vi "New Button Gallery.vi"(8 "Error In":errorcluster) -> (0 "Error Out":errorcluster, 3 "New Button Gallery":refnum<class "QWidget.lvclass">)   [LabVIEW 2014]
doc: "Dynamically assembles a widget that contains a variety of push buttons, checkboxes, and radio buttons. These buttons/checkboxes are grouped within group boxes.\n\nThe caller must manually make the returned widget visible.\n\n\nCopyright (c) 2019 Sze Howe Koh.\nThis code is licensed under the MIT license."
uses:
  <vilib>/addons/LQ/Qt Widgets/QWidget/QWidget.lvclass
  <vilib>/addons/LQ/Qt Widgets/QBoxLayout/Direction.ctl
  <vilib>/addons/LQ/Qt Widgets/QGroupBox/setCheckable.vi
  <vilib>/addons/LQ/Qt Widgets/QGroupBox/QGroupBox.lvclass
  <vilib>/addons/LQ/Qt Widgets/QPushButton/QPushButton.lvclass
  <vilib>/addons/LQ/Qt Widgets/QBoxLayout/QBoxLayout.lvclass
  <vilib>/addons/LQ/Qt Widgets/QCheckBox/QCheckBox.lvclass
  <vilib>/addons/LQ/Qt Widgets/QRadioButton/QRadioButton.lvclass
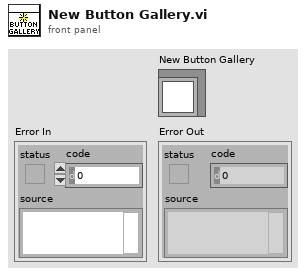
[diagram p1: front panel]
types:
  T1 = typedef "QBoxLayout.lvclass/Direction.ctl" = i32
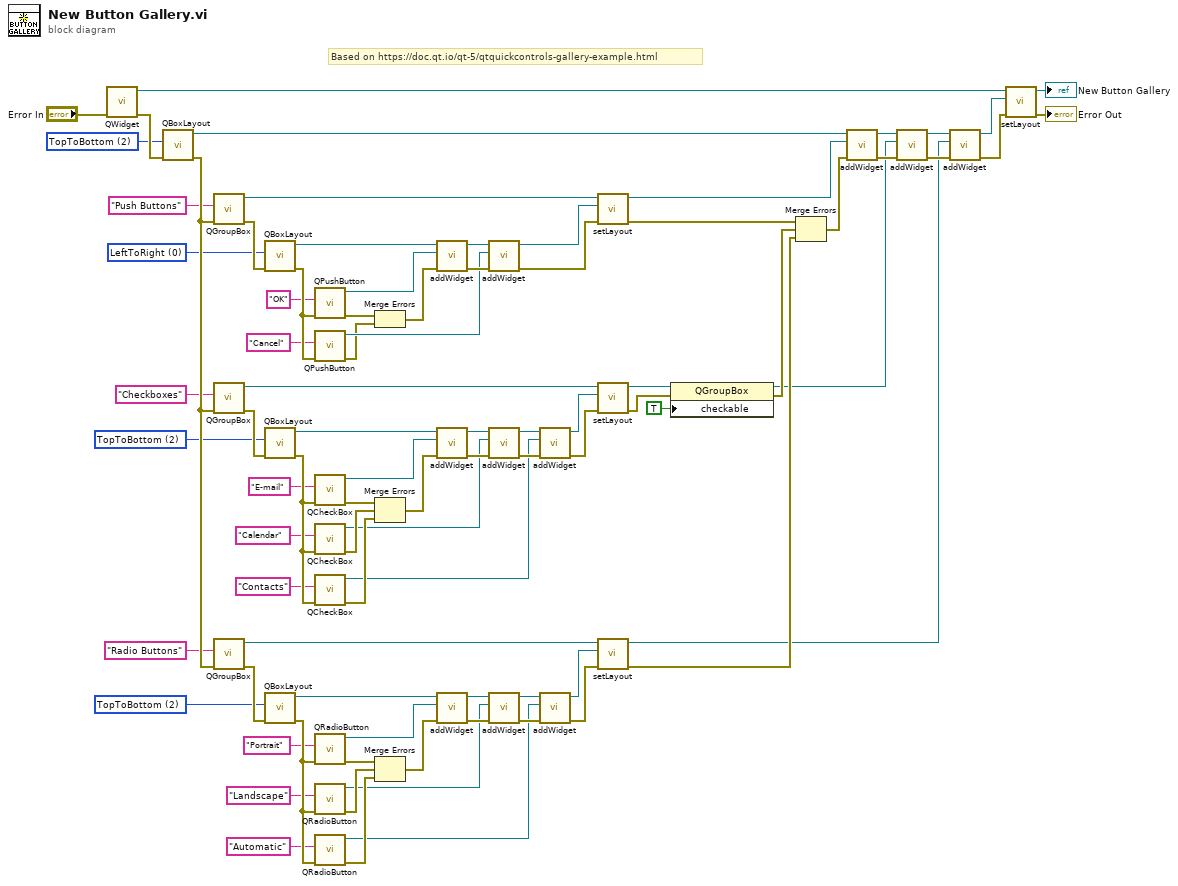
[diagram p0: block diagram]
diagram:
  w30 = T1 2 items=["LeftToRight", "RightToLeft", "TopToBottom", "BottomToTop"] ("direction")
  w44 = T1 2 items=["LeftToRight", "RightToLeft", "TopToBottom", "BottomToTop"] ("direction")
  w45 = T1 2 items=["LeftToRight", "RightToLeft", "TopToBottom", "BottomToTop"] ("direction")
  w46 = T1 0 items=["LeftToRight", "RightToLeft", "TopToBottom", "BottomToTop"] ("direction")
  # "Based on https://doc.qt.io/qt-5/qtquickcontrols-gallery-example.html"
  n1 = call <vilib>:"QWidget.vi"("Error In"="Error In") -> ("Error Out"=w83:errorcluster, "New QWidget"=w47:refnum<class "QWidget.lvclass">)  [unwired: 9 in]
  n2 = call <vilib>:"QBoxLayout.vi"("Error In"=w83, "direction"=w45) -> ("Error Out"=w75:errorcluster, "New QBoxLayout"=w49:refnum<class "QBoxLayout.lvclass">)  [unwired: 8 in]
  n3 = call <vilib>:"QGroupBox.vi"("Error In"=w75, "title"="Push Buttons") -> ("Error Out"=w84:errorcluster, "New QGroupBox"=w69:refnum<class "QGroupBox.lvclass">)  [unwired: 8 in]
  n4 = call <vilib>:"QGroupBox.vi"("Error In"=w75, "title"="Checkboxes") -> ("Error Out"=w77:errorcluster, "New QGroupBox"=w51:refnum<class "QGroupBox.lvclass">)  [unwired: 8 in]
  n5 = call <vilib>:"QGroupBox.vi"("Error In"=w75, "title"="Radio Buttons") -> ("Error Out"=w74:errorcluster, "New QGroupBox"=w14:refnum<class "QGroupBox.lvclass">)  [unwired: 8 in]
  n6 = call <vilib>:"QBoxLayout.vi"("Error In"=w84, "direction"=w46) -> ("Error Out"=w85:errorcluster, "New QBoxLayout"=w68:refnum<class "QBoxLayout.lvclass">)  [unwired: 8 in]
  n7 = call <vilib>:"QBoxLayout.vi"("Error In"=w77, "direction"=w44) -> ("Error Out"=w76:errorcluster, "New QBoxLayout"=w57:refnum<class "QBoxLayout.lvclass">)  [unwired: 8 in]
  n8 = call <vilib>:"QBoxLayout.vi"("Error In"=w74, "direction"=w30) -> ("Error Out"=w73:errorcluster, "New QBoxLayout"=w24:refnum<class "QBoxLayout.lvclass">)  [unwired: 8 in]
  n9 = call <vilib>:"QPushButton.vi"("Error In"=w85, "text"="OK") -> ("Error Out"=w42:errorcluster, "New QPushButton"=w66:refnum<class "QPushButton.lvclass">)  [unwired: 8 in]
  n10 = call <vilib>:"QPushButton.vi"("Error In"=w85, "text"="Cancel") -> ("Error Out"=w41:errorcluster, "New QPushButton"=w61:refnum<class "QPushButton.lvclass">)  [unwired: 8 in]
  n11 = call <vilib>:"QCheckBox.vi"("Error In"=w76, "text"="E-mail") -> ("Error Out"=w38:errorcluster, "New QCheckBox"=w54:refnum<class "QCheckBox.lvclass">)  [unwired: 8 in]
  n12 = call <vilib>:"QCheckBox.vi"("Error In"=w76, "text"="Calendar") -> ("Error Out"=w78:errorcluster, "New QCheckBox"=w53:refnum<class "QCheckBox.lvclass">)  [unwired: 8 in]
  n13 = call <vilib>:"QCheckBox.vi"("Error In"=w76, "text"="Contacts") -> ("Error Out"=w79:errorcluster, "New QCheckBox"=w52:refnum<class "QCheckBox.lvclass">)  [unwired: 8 in]
  n14 = call <vilib>:"QRadioButton.vi"("Error In"=w73, "text"="Portrait") -> ("Error Out"=w23:errorcluster, "New QRadioButton"=w19:refnum<class "QRadioButton.lvclass">)  [unwired: 8 in]
  n15 = call <vilib>:"QRadioButton.vi"("Error In"=w73, "text"="Landscape") -> ("Error Out"=w21:errorcluster, "New QRadioButton"=w16:refnum<class "QRadioButton.lvclass">)  [unwired: 8 in]
  n16 = call <vilib>:"QRadioButton.vi"("Error In"=w73, "text"="Automatic") -> ("Error Out"=w22:errorcluster, "New QRadioButton"=w15:refnum<class "QRadioButton.lvclass">)  [unwired: 8 in]
  n17 = Merge Errors(w42, w41) -> (w40:errorcluster)
  n18 = Merge Errors(w38, w78, w79) -> (w37:errorcluster)
  n19 = Merge Errors(w23, w21, w22) -> (w20:errorcluster)
  n20 = call <vilib>:"addWidget.vi"("Error In"=w40, "widget"=w66, "QBoxLayout In"=w68) -> ("Error Out"=w82:errorcluster, "QBoxLayout Out"=w67:refnum<class "QBoxLayout.lvclass">)  [unwired: 7 in]
  n21 = call <vilib>:"addWidget.vi"("Error In"=w37, "widget"=w54, "QBoxLayout In"=w57) -> ("Error Out"=w80:errorcluster, "QBoxLayout Out"=w56:refnum<class "QBoxLayout.lvclass">)  [unwired: 7 in]
  n22 = call <vilib>:"addWidget.vi"("Error In"=w20, "widget"=w19, "QBoxLayout In"=w24) -> ("Error Out"=w18:errorcluster, "QBoxLayout Out"=w25:refnum<class "QBoxLayout.lvclass">)  [unwired: 7 in]
  n23 = call <vilib>:"addWidget.vi"("Error In"=w82, "widget"=w61, "QBoxLayout In"=w67) -> ("Error Out"=w39:errorcluster, "QBoxLayout Out"=w65:refnum<class "QBoxLayout.lvclass">)  [unwired: 7 in]
  n24 = call <vilib>:"addWidget.vi"("Error In"=w80, "widget"=w53, "QBoxLayout In"=w56) -> ("Error Out"=w81:errorcluster, "QBoxLayout Out"=w55:refnum<class "QBoxLayout.lvclass">)  [unwired: 7 in]
  n25 = call <vilib>:"addWidget.vi"("Error In"=w18, "widget"=w16, "QBoxLayout In"=w25) -> ("Error Out"=w17:errorcluster, "QBoxLayout Out"=w26:refnum<class "QBoxLayout.lvclass">)  [unwired: 7 in]
  n26 = call <vilib>:"addWidget.vi"("Error In"=w81, "widget"=w52, "QBoxLayout In"=w55) -> ("Error Out"=w36:errorcluster, "QBoxLayout Out"=w50:refnum<class "QBoxLayout.lvclass">)  [unwired: 7 in]
  n27 = call <vilib>:"addWidget.vi"("Error In"=w17, "widget"=w15, "QBoxLayout In"=w26) -> ("Error Out"=w12:errorcluster, "QBoxLayout Out"=w13:refnum<class "QBoxLayout.lvclass">)  [unwired: 7 in]
  n28 = call <vilib>:"setLayout.vi"("Error In"=w39, "layout"=w65, "QWidget In"=w69) -> ("Error Out"=w2:errorcluster, "QWidget Out"=w3:refnum<class "QGroupBox.lvclass">)  [unwired: 7 in]
  n29 = call <vilib>:"setLayout.vi"("Error In"=w36, "layout"=w50, "QWidget In"=w51) -> ("Error Out"=w6:errorcluster, "QWidget Out"=w7:refnum<class "QGroupBox.lvclass">)  [unwired: 7 in]
  n30 = call <vilib>:"setLayout.vi"("Error In"=w12, "layout"=w13, "QWidget In"=w14) -> ("Error Out"=w72:errorcluster, "QWidget Out"=w1:refnum<class "QGroupBox.lvclass">)  [unwired: 7 in]
  n31 = property class="QGroupBox"(reference=w7, error in=w6, "checkable"=TRUE) -> (reference out=w5:refnum<class "QGroupBox.lvclass">, error out=w71:errorcluster)
  n32 = Merge Errors(w2, w71, w72) -> (w33:errorcluster)
  n33 = call <vilib>:"addWidget.vi"("Error In"=w33, "widget"=w3, "QBoxLayout In"=w49) -> ("Error Out"=w32:errorcluster, "QBoxLayout Out"=w48:refnum<class "QBoxLayout.lvclass">)  [unwired: 7 in]
  n34 = call <vilib>:"addWidget.vi"("Error In"=w32, "widget"=w5, "QBoxLayout In"=w48) -> ("Error Out"=w9:errorcluster, "QBoxLayout Out"=w11:refnum<class "QBoxLayout.lvclass">)  [unwired: 7 in]
  n35 = call <vilib>:"addWidget.vi"("Error In"=w9, "widget"=w1, "QBoxLayout In"=w11) -> ("Error Out"=w8:errorcluster, "QBoxLayout Out"=w10:refnum<class "QBoxLayout.lvclass">)  [unwired: 7 in]
  n36 = call <vilib>:"setLayout.vi"("Error In"=w8, "layout"=w10, "QWidget In"=w47) -> ("Error Out"=→"Error Out":errorcluster, "QWidget Out"=→"New Button Gallery":refnum<class "QWidget.lvclass">)  [unwired: 7 in]
